vi "Configure Ramp.vi"(6 "Rate Value (0.001)":dbl=0.001 min=0.001 max=100.0 step=0.001 format="%.3f", 8 "error in (no error)":errorcluster, 9 "Enable Ramping (F: Disable)":bool, 10 "Output (0: Sample Heater)":u16(ring) items=["Sample Heater ", "Warm-up Heater "], 11 "VISA resource name":refnum<visa-resource-name>) -> (0 "error out":errorcluster, 3 "VISA resource name out":refnum<visa-resource-name>)   [LabVIEW 2018, in "Lake Shore 372.lvlib"]
doc: "Configures the parameters of setpoint ramp."
uses:
  Lake Shore 372.lvlib
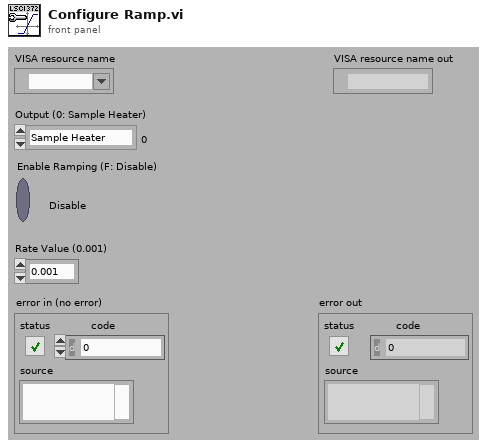
[diagram p1: front panel]
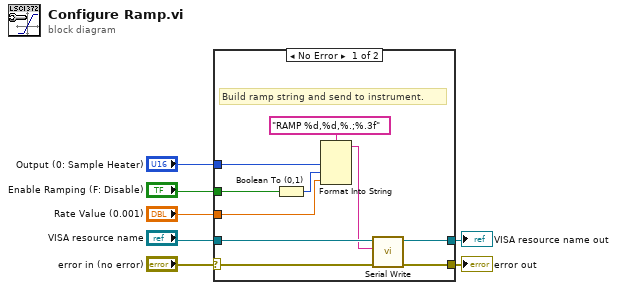
[diagram p0: block diagram]
diagram:
  n1 = case shown="No Error" "error in (no error)" {
    selector: "error in (no error)" -> [w8 w18]
    tunnel: "Enable Ramping (F: Disable)" -> [w17 _]
    tunnel: "VISA resource name" -> [w16 w19]
    tunnel: [w15 w18] -> w5
    tunnel: [w14 w19] -> w4
    tunnel: "Output (0: Sample Heater)" -> [w12 _]
    tunnel: "Rate Value (0.001)" -> [w10 _]
    frame No Error {
      # "Build ramp string and send to instrument."
      n2 = Boolean To (0,1)(Boolean=w17) -> (0, 1=w11:i16)
      n3 = Format Into String(format string="RAMP %d,%d,%.;%.3f", w12, w11, w10) -> (resulting string=w9:string)  [unwired: 2 in, 1 out]
      n4 = call "Serial Write.vi"("error in (no error)"=w8, "Write Buffer (\"\")"=w9, "VISA resource name"=w16) -> ("error out"=w15:errorcluster, "VISA resource name out"=w14:refnum<visa-resource-name>)  [unwired: 6 in, 1 out]
    }
    frame Error {
    }
  }
  "error out" <- w5
  "VISA resource name out" <- w4
